vi "Get topic.vi"(11 "Unsubscribe JSON in":refnum<class "Unsubscribe JSON.lvclass">) -> (2 "Topic URl":string, 3 "Unsubscribe JSON out":refnum<class "Unsubscribe JSON.lvclass">)   [LabVIEW 2020, in "wamplv.lvlib" / "Unsubscribe JSON.lvclass"]
uses:
  Unsubscribe JSON.lvclass
  Unsubscribe JSON.lvclass/Unsubscribe JSON.ctl
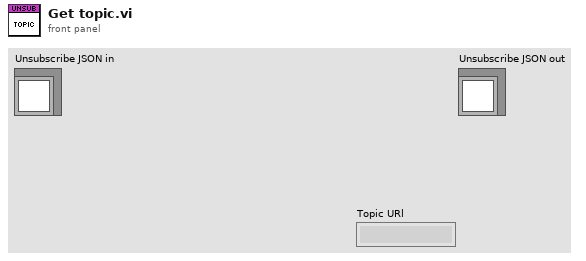
[diagram p1: front panel]
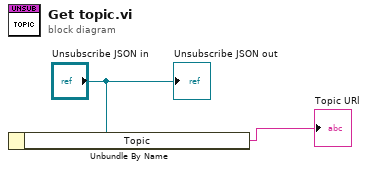
[diagram p0: block diagram]
diagram:
  n1 = Unbundle By Name("Unsubscribe JSON in") -> ("Topic"=→"Topic URl":string)
  "Unsubscribe JSON out" <- "Unsubscribe JSON in"
